vi "Position VLC Window.vi"(8 "error in (no error)":errorcluster, 10 "Main Tab Ref":refnum<vi>, 11 "VLC Ref":refnum<vi>) -> (0 "error out":errorcluster)   [LabVIEW 2014]
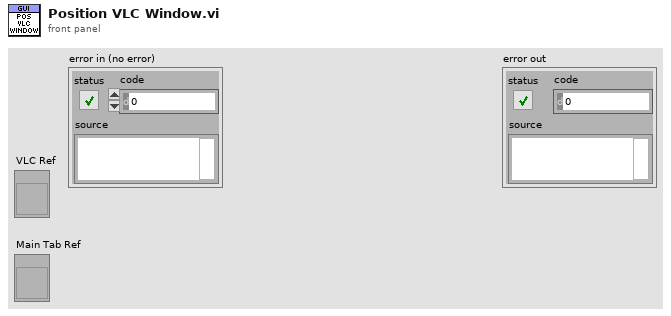
[diagram p1: front panel]
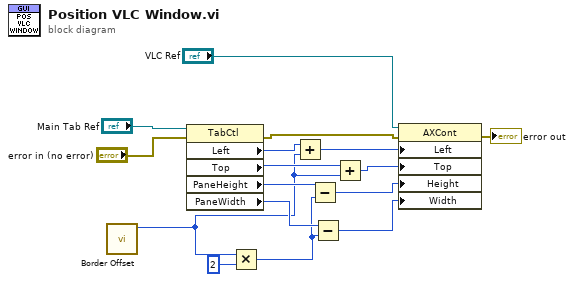
[diagram p0: block diagram]
diagram:
  n1 = call "Border Offset.vi"() -> ("Border Offset (px)"=w1:i32)  [unwired: 11 in]
  n2 = property class="TabCtl"(reference="Main Tab Ref", error in="error in (no error)") -> (error out=w4:errorcluster, "Left"=w8:i32, "Top"=w7:i32, "PaneHeight"=w15:u32, "PaneWidth"=w14:u32)  [unwired: 1 out]
  n3 = Multiply(x=w1, y=u32 2) -> (x*y=w12:u32)
  n4 = Add(x=w8, y=w1) -> (x+y=w5:i32)
  n5 = Subtract(x=w15, y=w12) -> (x-y=w11:u32)
  n6 = Subtract(x=w14, y=w12) -> (x-y=w10:u32)
  n7 = Add(x=w7, y=w1) -> (x+y=w6:i32)
  n8 = property class="AXCont"(reference="VLC Ref", error in=w4, "Left"=w5, "Top"=w6, "Height"=w11, "Width"=w10) -> (error out=→"error out":errorcluster)  [unwired: 1 out]
